vi "channeldata_digitalwfm.vi"() -> ()   [LabVIEW 2019]
panel:
  out "Error Out":errorcluster
  in  "TDMS File":path=path "C:/Python/projects/nitdms/tests/tdms_files/channeldata_digitalwfm.tdms"
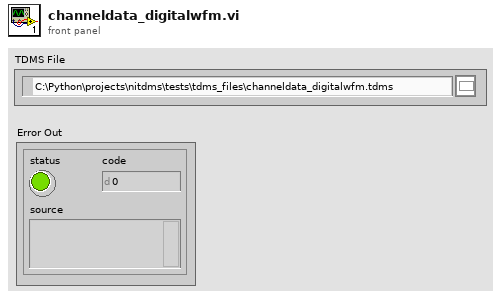
[diagram p1: front panel]
types:
  T1 = enum16{"open", "open or create", "create or replace", "create", "open (read-only)"}
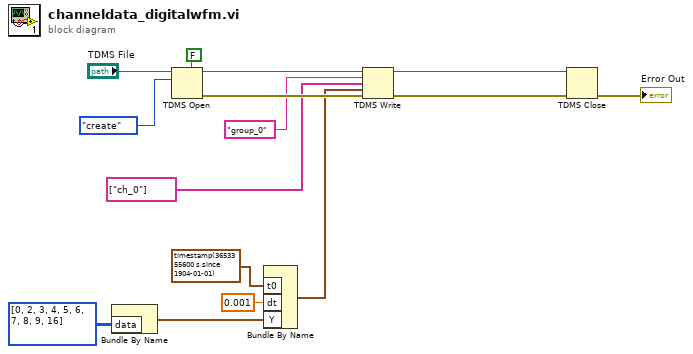
[diagram p0: block diagram]
diagram:
  n1 = Bundle By Name("data"=u8[][] [[0], [2], [3], [4], [5], [6], [7], [8], [9], [16]]) -> (w10:digitaldata)  [unwired: 1 in]
  n2 = TDMS Open(5:FALSE ("create index file? (T)"), 10:T1."create" ("operation (0:open)"), 11:"TDMS File") -> (0:w7:errorcluster, 3:w6:refnum<k34>)  [unwired: 4 in]
  n3 = Bundle By Name("t0"=timestamp(3653355600 s since 1904-01-01), "dt"=0.001, "Y"=w10) -> (w2:digitalwaveform)  [unwired: 1 in]
  n4 = TDMS Write(0:w6, 5:"group_0", 7:string[] ["ch_0"], 9:w2, 11:w7) -> (4:w4:refnum<k34>, 15:w5:errorcluster)  [unwired: 1 in, 2 out]
  n5 = TDMS Close(8:w5, 11:w4) -> (0:→"Error Out":errorcluster)  [unwired: 1 out]
